vi "Practica 11 - Icono SubPrograma.vi"() -> ()   [LabVIEW 2021]
panel:
  out "Boolean 2":bool
  out "Fahrenheit":dbl
  out "Centigrado":dbl
  in  "Entrada":dbl
  in  "Boolean":bool
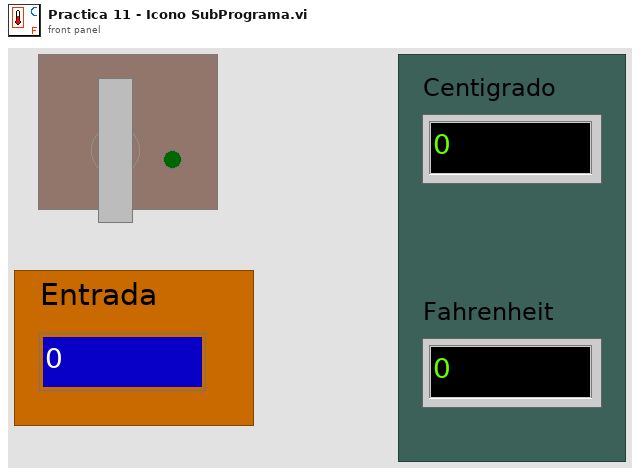
[diagram p1: front panel]
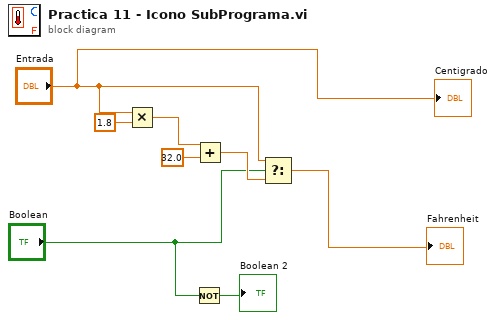
[diagram p0: block diagram]
diagram:
  n1 = Multiply(x="Entrada", y=1.8) -> (x*y=w7:dbl)
  n2 = Not(x="Boolean") -> (.not. x?=→"Boolean 2":bool)
  n3 = Add(x=w7, y=32.0) -> (x+y=w5:dbl)
  n4 = Select(t="Entrada", s="Boolean", f=w5) -> (s? t:f=→"Fahrenheit":dbl)
  "Centigrado" <- "Entrada"
